vi "Disable Routing Channel.vi"(8 "error in":errorcluster, 11 "routing channel in":T1 format="%.0x") -> (0 "error out":errorcluster, 3 "routing channel out":T1 format="%.0x")   [LabVIEW 2020, in "Routing and Faulting Scripting.lvlib"]
doc: "Disables a routing channel. Disabled channels are not accessible while deployed."
uses:
  Routing and Faulting Scripting.lvlib
  <vilib>/NI VeriStand/Custom Device API/Custom Device Item Ref.ctl
  <vilib>/NI VeriStand/Custom Device API/Custom Device API.lvlib
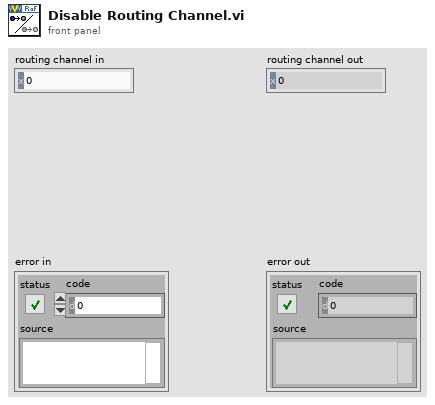
[diagram p1: front panel]
types:
  T1 = typedef "Custom Device API.lvlib/Custom Device Item Ref.ctl" = u64
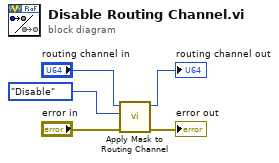
[diagram p0: block diagram]
diagram:
  n1 = call "Apply Mask to Routing Channel.vi"("error in"="error in", "mask"=enum16{"Disable", "Enable"}."Disable" ("Mask"), "routing channel in"="routing channel in") -> ("error out"=→"error out":errorcluster, "routing channel out"=→"routing channel out":T1)  [unwired: 7 in]
